vi "Get Value.vi"(8 "error in (no error)":errorcluster, 11 "Variant Value Source in":refnum<class "Variant Value Source.lvclass">) -> (0 "error out":errorcluster, 2 "Value":variant, 3 "Variant Value Source out":refnum<class "Variant Value Source.lvclass">)   [LabVIEW 2020, in "Composed Columns.lvlib" / "Variant Value Source.lvclass"]
uses:
  Variant Value Source.lvclass
  Variant Value Source.lvclass/Variant Value Source.ctl
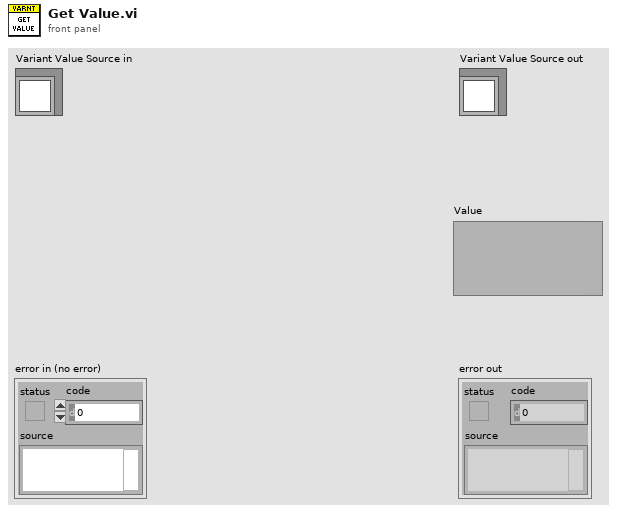
[diagram p1: front panel]
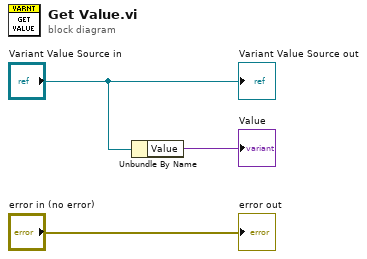
[diagram p0: block diagram]
diagram:
  n1 = Unbundle By Name("Variant Value Source in") -> ("Value"=→"Value":variant)
  "error out" <- "error in (no error)"
  "Variant Value Source out" <- "Variant Value Source in"
